vi "RSNRPZ Sensor Info.vi"(7 "Array Size (100)":i32=100, 8 "error in (no error)":errorcluster, 9 "Info Type (\"\")":string, 10 "Channel (1)":i32=1, 11 "VISA session":refnum<visa-resource-name> caption="VISA resource name") -> (0 "error out":errorcluster, 2 "Info":string, 3 "dup VISA session":refnum<visa-resource-name> caption="VISA resource name")   [LabVIEW 2010]
doc: "This VI returns selected information on a sensor.\n\nRemote-control command(s):\nSYST:INFO? <Info Type>"
uses:
  rsnrpz_32.dll
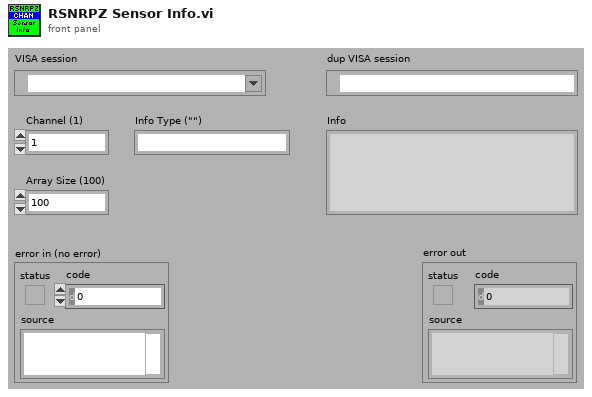
[diagram p1: front panel]
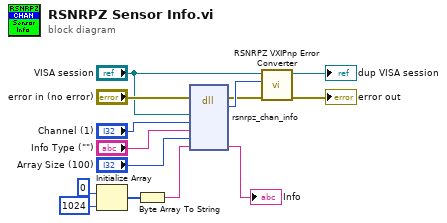
[diagram p0: block diagram]
diagram:
  n1 = Initialize Array(u8 0, 1024) -> (w12:u8[])
  n2 = Byte Array To String(unsigned byte array=w12) -> (string=w7:string)
  n3 = dll-call lib="rsnrpz_32.dll" fn="rsnrpz_chan_info"(error in="error in (no error)", "Instrument Handle"="VISA session", "Channel"="Channel (1)", "Info Type"="Info Type (\"\")", "Array Size"="Array Size (100)", "Info"=w7) -> (error out=w5:errorcluster, "Status"=w11:i32, "Info"=→"Info":string)  [unwired: 6 in, 1 out]
  n4 = call <instrlib>:"RSNRPZ VXIPnp Error Converter.vi"("error in"=w5, "VXIPnp error code"=w11, "VISA session"="VISA session") -> ("error out"=→"error out":errorcluster, "dup VISA session"=→"dup VISA session":refnum<visa-resource-name>)  [unwired: 7 in]
